vi "关键参数转u16数组.vi"(11 "关键参数":T1(array[cluster])) -> (3 "添加的数组":u16[](array[numeric]))   [LabVIEW 2016, in "MB SLAVE.lvlib"]
uses:
  MB SLAVE.lvlib
panel:
  out "大小":i32
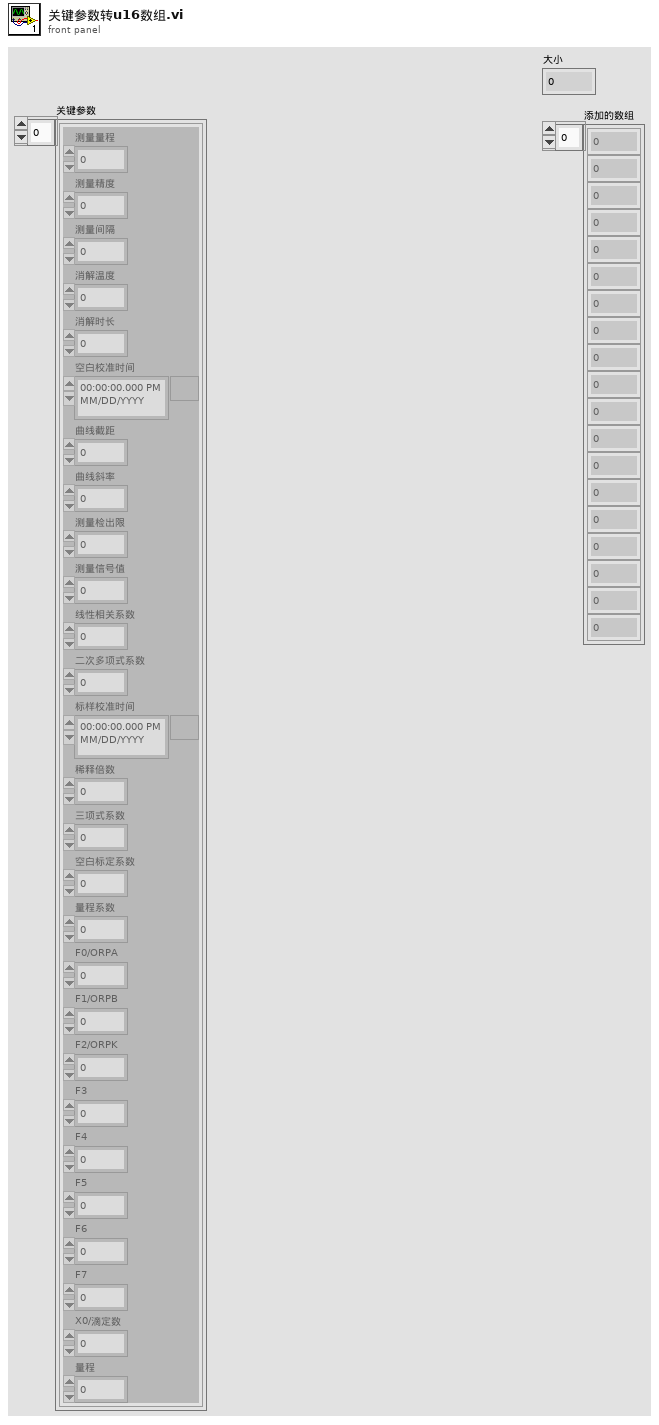
[diagram p1: front panel]
types:
  T1 = cluster{"测量量程":dbl, "测量精度":dbl, "测量间隔":dbl, "消解温度":dbl, "消解时长":dbl, "空白校准时间":timestamp, "曲线截距":dbl, "曲线斜率":dbl, "测量检出限":dbl, "测量信号值":dbl, "线性相关系数":dbl, "二次多项式系数":dbl, "标样校准时间":timestamp, "稀释倍数":dbl, "三项式系数":dbl, "空白标定系数":dbl, "量程系数":dbl, "F0/ORPA":dbl, "F1/ORPB":dbl, "F2/ORPK":dbl, "F3":dbl, "F4":dbl, "F5":dbl, "F6":dbl, "F7":dbl, "X0/滴定数":dbl, "量程":dbl}[]
  T2 = cluster{"测量量程":dbl, "测量精度":dbl, "测量间隔":dbl, "消解温度":dbl, "消解时长":dbl, "空白校准时间":timestamp, "曲线截距":dbl, "曲线斜率":dbl, "测量检出限":dbl, "测量信号值":dbl, "线性相关系数":dbl, "二次多项式系数":dbl, "标样校准时间":timestamp, "稀释倍数":dbl, "三项式系数":dbl, "空白标定系数":dbl, "量程系数":dbl, "F0/ORPA":dbl, "F1/ORPB":dbl, "F2/ORPK":dbl, "F3":dbl, "F4":dbl, "F5":dbl, "F6":dbl, "F7":dbl, "X0/滴定数":dbl, "量程":dbl}
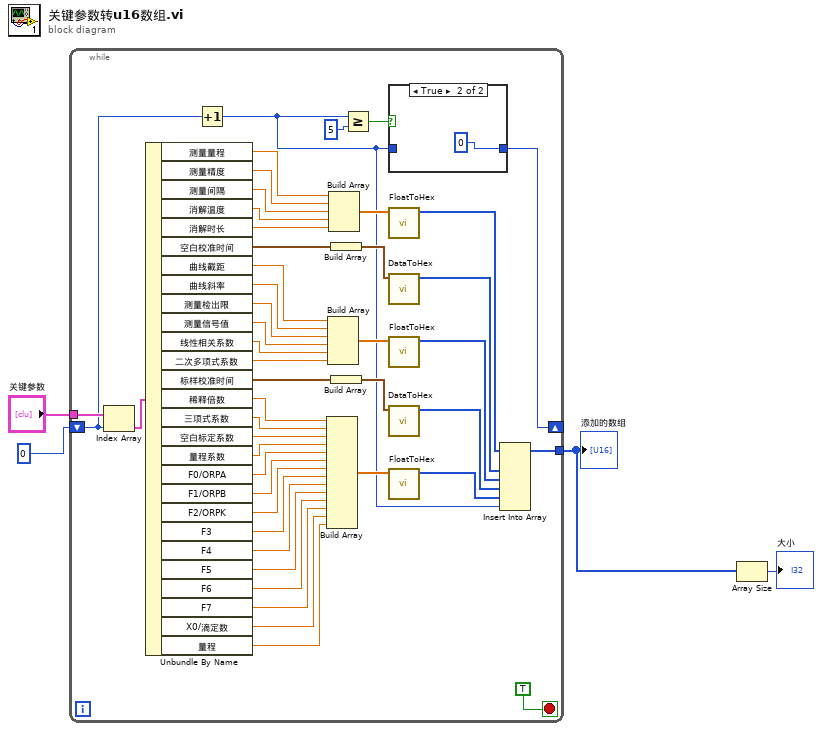
[diagram p0: block diagram]
diagram:
  n1 = while {
    tunnel: "关键参数" -> [w13]
    shift-right: [w6] -> _
    shift-left: 0 -> [w10]
    tunnel: [w9] -> w2
    stop <- TRUE stop-if-true
    n2 = Index Array(array=w13, index=w10) -> (element=w12:T2)
    n3 = Unbundle By Name(w12) -> ("测量量程"=w50:dbl, "测量精度"=w48:dbl, "测量间隔"=w47:dbl, "消解温度"=w46:dbl, "消解时长"=w45:dbl, "空白校准时间"=w44:timestamp, "曲线截距"=w42:dbl, "曲线斜率"=w41:dbl, "测量检出限"=w40:dbl, "测量信号值"=w39:dbl, "线性相关系数"=w38:dbl, "二次多项式系数"=w37:dbl, "标样校准时间"=w36:timestamp, "稀释倍数"=w34:dbl, "三项式系数"=w33:dbl, "空白标定系数"=w32:dbl, "量程系数"=w31:dbl, "F0/ORPA"=w30:dbl, "F1/ORPB"=w29:dbl, "F2/ORPK"=w28:dbl, "F3"=w27:dbl, "F4"=w26:dbl, "F5"=w25:dbl, "F6"=w24:dbl, "F7"=w23:dbl, "X0/滴定数"=w22:dbl, "量程"=w21:dbl)
    n4 = Increment(x=w10) -> (x+1=w5:i32)
    n5 = Build Array(w34, w33, w32, w31, w30, w29, w28, w27, w26, w25, w24, w23, w22, w21) -> (w20:dbl[])
    n6 = Build Array(w42, w41, w40, w39, w38, w37) -> (w19:dbl[])
    n7 = Build Array(w50, w48, w47, w46, w45) -> (w49:dbl[])
    n8 = Build Array(w44) -> (w43:timestamp[])
    n9 = Build Array(w36) -> (w35:timestamp[])
    n10 = Greater Or Equal?(x=w5, y=u16 5) -> (x >= y?=w7:bool)
    n11 = case shown="True" w7 {
      tunnel: [w51 u16 0] -> w6
      tunnel: w5 -> [w51 _]
      frame False {
      }
      frame True {
      }
    }
    n12 = call "FloatToHex.vi"("FLOAT"=w49) -> ("交织的数组"=w18:u16[])  [unwired: 10 in]
    n13 = call "DataToHex.vi"("time"=w43) -> ("数组"=w17:u16[])  [unwired: 10 in]
    n14 = call "FloatToHex.vi"("FLOAT"=w19) -> ("交织的数组"=w16:u16[])  [unwired: 10 in]
    n15 = call "DataToHex.vi"("time"=w35) -> ("数组"=w15:u16[])  [unwired: 10 in]
    n16 = call "FloatToHex.vi"("FLOAT"=w20) -> ("交织的数组"=w14:u16[])  [unwired: 10 in]
    n17 = Insert Into Array(array=w18, new element #1=w17, new element #2=w16, new element #3=w15, new element #4=w14, new element #5=w5) -> (w9:u16[])  [unwired: 1 in]
  }
  "添加的数组" <- w2
  n18 = Array Size(array=w2) -> (size(s)=→"大小":i32)
